vi "Post Iterate.vi"(8 "error in (no error)":errorcluster, 11 "Example Actor in":refnum<class "Example Actor.lvclass">) -> (0 "error out":errorcluster, 3 "Example Actor out":refnum<class "Example Actor.lvclass">)   [LabVIEW 2023, in "Example Iterator NR Actor Auto Iteration Notification.lvlib" / "Example Actor.lvclass"]
doc: "Method called after the iterations"
uses:
  Example Actor.lvclass
  Example Actor.lvclass/Example Actor.ctl
  <userlib>/_OpenG.lib/time/time.llb/openg_time.lvlib
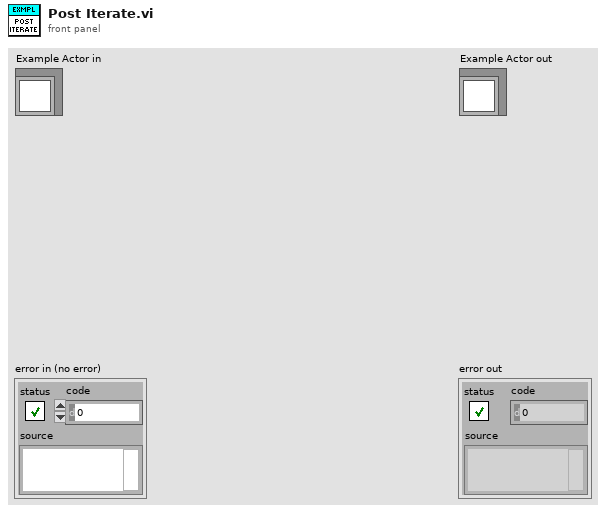
[diagram p1: front panel]
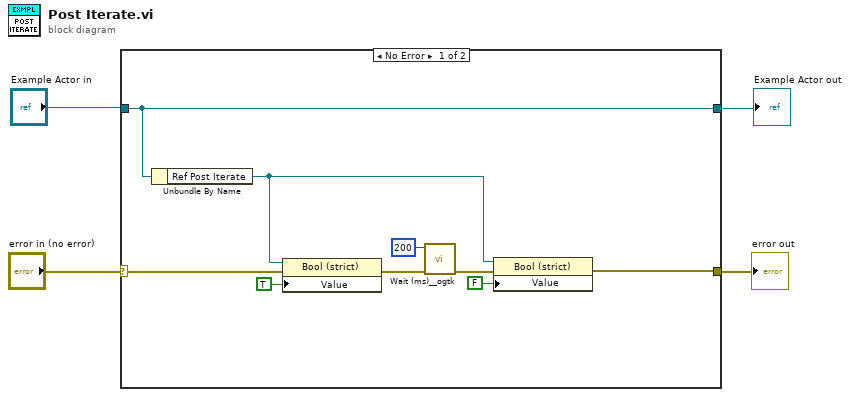
[diagram p0: block diagram]
diagram:
  n1 = case shown="No Error" "error in (no error)" {
    selector: "error in (no error)" -> [w12 w15]
    tunnel: [w5 w15] -> w1
    tunnel: [w13 w14] -> w3
    tunnel: "Example Actor in" -> [w13 w14]
    frame No Error {
      n2 = Unbundle By Name(w13) -> ("Ref Post Iterate"=w9:refnum<vi>)
      n3 = property class="Bool (strict)"(reference=w9, error in=w12, "Value"=TRUE) -> (error out=w11:errorcluster)  [unwired: 1 out]
      n4 = call <userlib>:"Wait (ms)__ogtk.vi"("error in (no error)"=w11, "milliseconds to wait"=u32 200) -> ("error out"=w10:errorcluster)  [unwired: 8 in, 1 out]
      n5 = property class="Bool (strict)"(reference=w9, error in=w10, "Value"=FALSE) -> (error out=w5:errorcluster)  [unwired: 1 out]
    }
    frame Error {
    }
  }
  "error out" <- w1
  "Example Actor out" <- w3
